vi "Drive Distance.vi"(11 "Desired Distance":dbl) -> (3 "Done?":bool)   [LabVIEW 2016]
uses:
  Robot Values.vi
  <vilib>/addons/control/pid/pid.llb/PID (DBL).vi
  <vilib>/addons/control/pid/NI_PID_pid.lvlib
panel:
  in  "Error PID gains":T1={"proportional gain (Kc)"=1.0, "integral time (Ti, min)"=0.01, "derivative time (Td, min)"=0.0} {"derivative time (Td, min)" format="%.3f"; "integral time (Ti, min)" format="%.3f"; "proportional gain (Kc)" format="%.3f"}
  in  "Distance PID gains":T1={"proportional gain (Kc)"=1.0, "integral time (Ti, min)"=0.01, "derivative time (Td, min)"=0.0} {"derivative time (Td, min)" format="%.3f"; "integral time (Ti, min)" format="%.3f"; "proportional gain (Kc)" format="%.3f"}
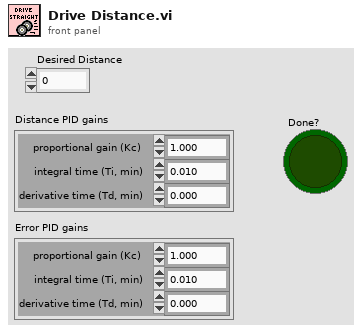
[diagram p1: front panel]
types:
  T1 = cluster{"proportional gain (Kc)":dbl, "integral time (Ti, min)":dbl, "derivative time (Td, min)":dbl}
  T2 = typedef "Robot Values.ctl" = cluster{"Robot Drive":cluster{"Left Motor Power":dbl, "Right Motor Power":dbl, "Left Encoder Value":dbl, "Right Encoder Value":dbl}, "Sensors":cluster{"Gyro Angle":dbl, "Recalibrate Gyro":bool, "Reset Gyro":bool}, "Climbing":cluster{"Climber State":bool, "Gear State":dbl}, "Shooter":cluster{"Shooter Wheels":bool}, "Conveyor":cluster{"Conveyor State":bool}, "Robot States":cluster{"Drive mode":string}}
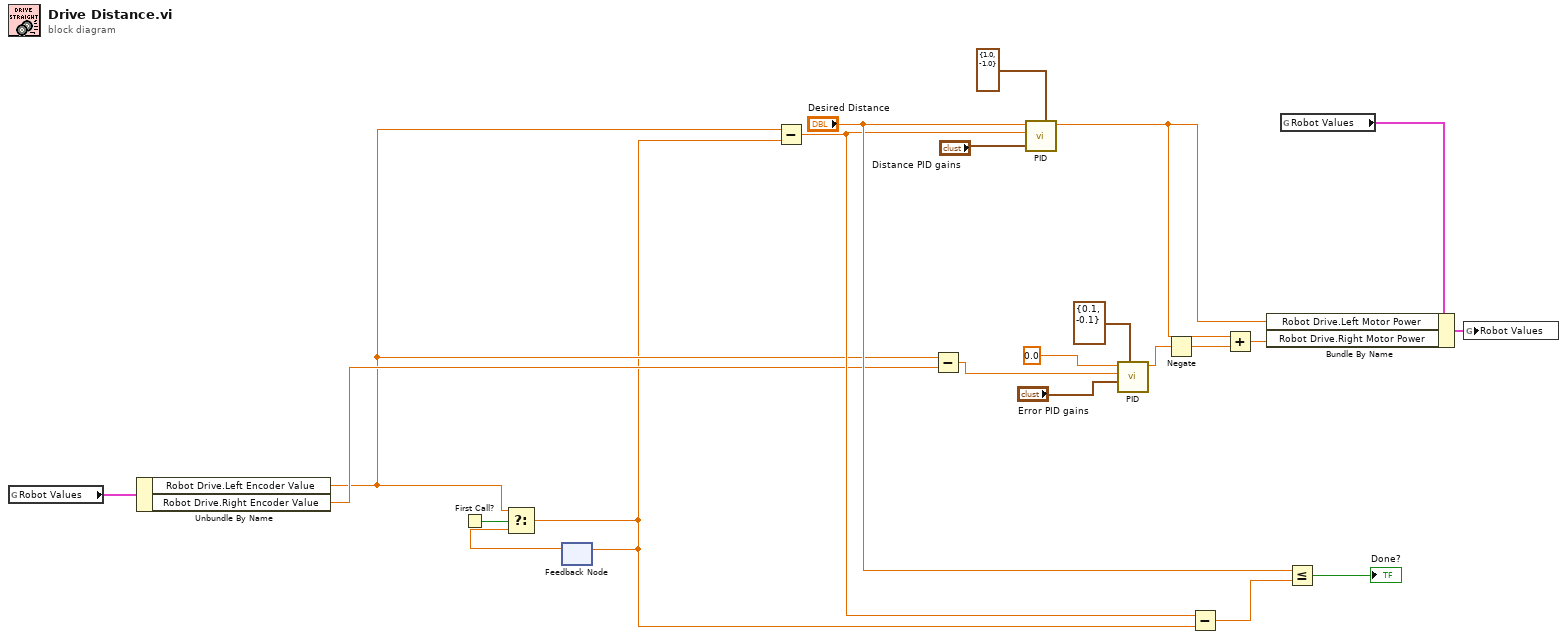
[diagram p0: block diagram]
diagram:
  n1 = global read "Robot Values.vi" "Robot Values"() -> (w22:T2)
  n2 = Unbundle By Name(w22) -> ("Robot Drive.Left Encoder Value"=w3:dbl, "Robot Drive.Right Encoder Value"=w8:dbl)
  n3 = First Call?() -> (First Call?: T/F=w4:bool)
  n4 = feedback #1() -> (w2:dbl)  [unwired: 1 in]
  n5 = Select(t=w3, s=w4, f=w2) -> (s? t:f=w1:dbl)
  n6 = feedback-in #1(w1) -> ()
  n7 = Subtract(x=w3, y=w1) -> (x-y=w9:dbl)
  n8 = Subtract(x=w3, y=w8) -> (x-y=w7:dbl)
  n9 = call-poly <vilib>:"PID.vi"("output range"=cluster{"output high":dbl, "output low":dbl} {"output high"=1.0, "output low"=-1.0}, "PID gains"="Distance PID gains", "process variable"=w9, "setpoint"="Desired Distance") -> ("output"=w11:dbl)  [unwired: 6 in, 1 out]
  n10 = call-poly <vilib>:"PID.vi"("output range"=cluster{"output high":dbl, "output low":dbl} {"output high"=0.1, "output low"=-0.1}, "PID gains"="Error PID gains", "process variable"=w7, "setpoint"=0.0) -> ("output"=w15:dbl)  [unwired: 6 in, 1 out]
  n11 = Negate(x=w15) -> (-x=w5:dbl)
  n12 = Subtract(x=w9, y=w1) -> (x-y=w10:dbl)
  n13 = Add(x=w11, y=w5) -> (x+y=w16:dbl)
  n14 = global read "Robot Values.vi" "Robot Values"() -> (w18:T2)
  n15 = Bundle By Name(cluster=w18, "Robot Drive.Left Motor Power"=w11, "Robot Drive.Right Motor Power"=w16) -> (w19:T2)
  n16 = Less Or Equal?(x="Desired Distance", y=w10) -> (x <= y?=→"Done?":bool)
  n17 = global write "Robot Values.vi" "Robot Values"(w19) -> ()
